vi "ComputeAddSize.vi"(1 "B Position":i32, 2 "B Array Size":i32, 3 "A Position":i32, 4 "A Array Size":i32) -> (0 "Digits":i32)   [LabVIEW 2025]
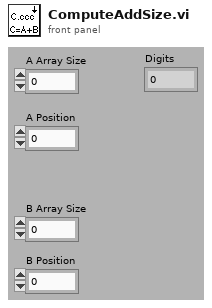
[diagram p1: front panel]
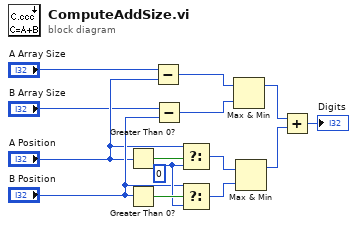
[diagram p0: block diagram]
diagram:
  w12 = 0
  n1 = Greater Than 0?(x="A Position") -> (x > 0?=w14:bool)
  n2 = Greater Than 0?(x="B Position") -> (x > 0?=w13:bool)
  n3 = Subtract(x="A Array Size", y="A Position") -> (x-y=w9:i32)
  n4 = Subtract(x="B Array Size", y="B Position") -> (x-y=w8:i32)
  n5 = Select(t="A Position", s=w14, f=w12) -> (s? t:f=w3:i32)
  n6 = Select(t="B Position", s=w13, f=w12) -> (s? t:f=w4:i32)
  n7 = Max & Min(x=w9, y=w8) -> (max(x,y)=w11:i32)  [unwired: 1 out]
  n8 = Max & Min(x=w3, y=w4) -> (max(x,y)=w5:i32)  [unwired: 1 out]
  n9 = Add(x=w11, y=w5) -> (x+y=→"Digits":i32)
